vi "ClassPanel.vi"(8 "error in (no error)":errorcluster caption="entrée d'erreur (pas d'erreur)", 11 "E8267D.lvclass":refnum<class "E8267D.lvclass">) -> (0 "error out":errorcluster caption="sortie d'erreur", 3 "E8267D.lvclass Out":refnum<class "E8267D.lvclass">)   [LabVIEW 2019, in "E8267D.lvclass"]
uses:
  E8267D.lvclass
  C:/Programmes Labview/LabscanV1A/DevicesClass/BaseDevice/BaseDevice.lvclass
  BaseDevice/ClassQueueMess.ctl
  E8267D_Func.ctl
  E8267D.lvclass/E8267D.ctl
  BaseDevice/Accessor/GetClassEvent.vi
panel:
  in  "PulseMode En":bool
  in  "Mod En":bool
  in  "Scan Mode":u16(ring) items=["Frequency", "Power"]
  in  "Output En":bool
  in  "Con/Disc.":bool
  in  "FUnits":u16(ring) caption="Units" items=["Hz", "MHz", "GHz"]
  in  "MainProgQ":refnum<queue>
  in  "MainProgQEvent":refnum<user-event>
  in  "Acq":bool
  in  "Stop":bool
  in  "Power":dbl caption="Power(dBm)" format="%#.3f"
  in  "MiseAJour":bool
  in  "Freq(Hz)":dbl=60.0 min=0.01 max=20500000000.0 step=0.01 format="%^#.5e"
  out "Init Program":bool
  # "PSG E8267D"
  # "this MUST labeled with class name"
  # "this MUST be present and labeled \"Stop\" and \"Acq\""
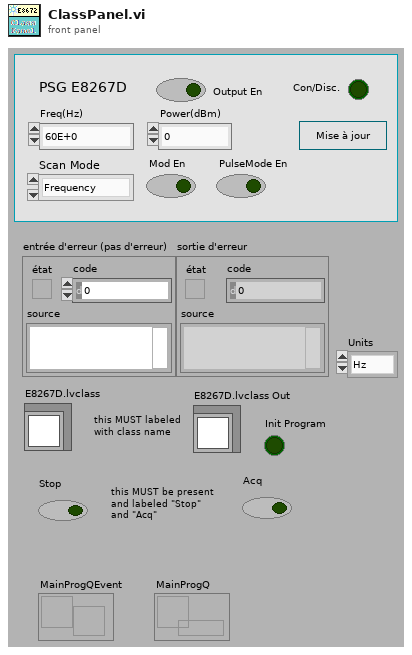
[diagram p1: front panel]
types:
  T1 = typedef "E8267D.lvclass/E8267D_Func.ctl" = enum16{"SetPower (dBm)", "SetFrequency (Hz)"}
  T2 = typedef "ClassQueueMess.ctl" = u16
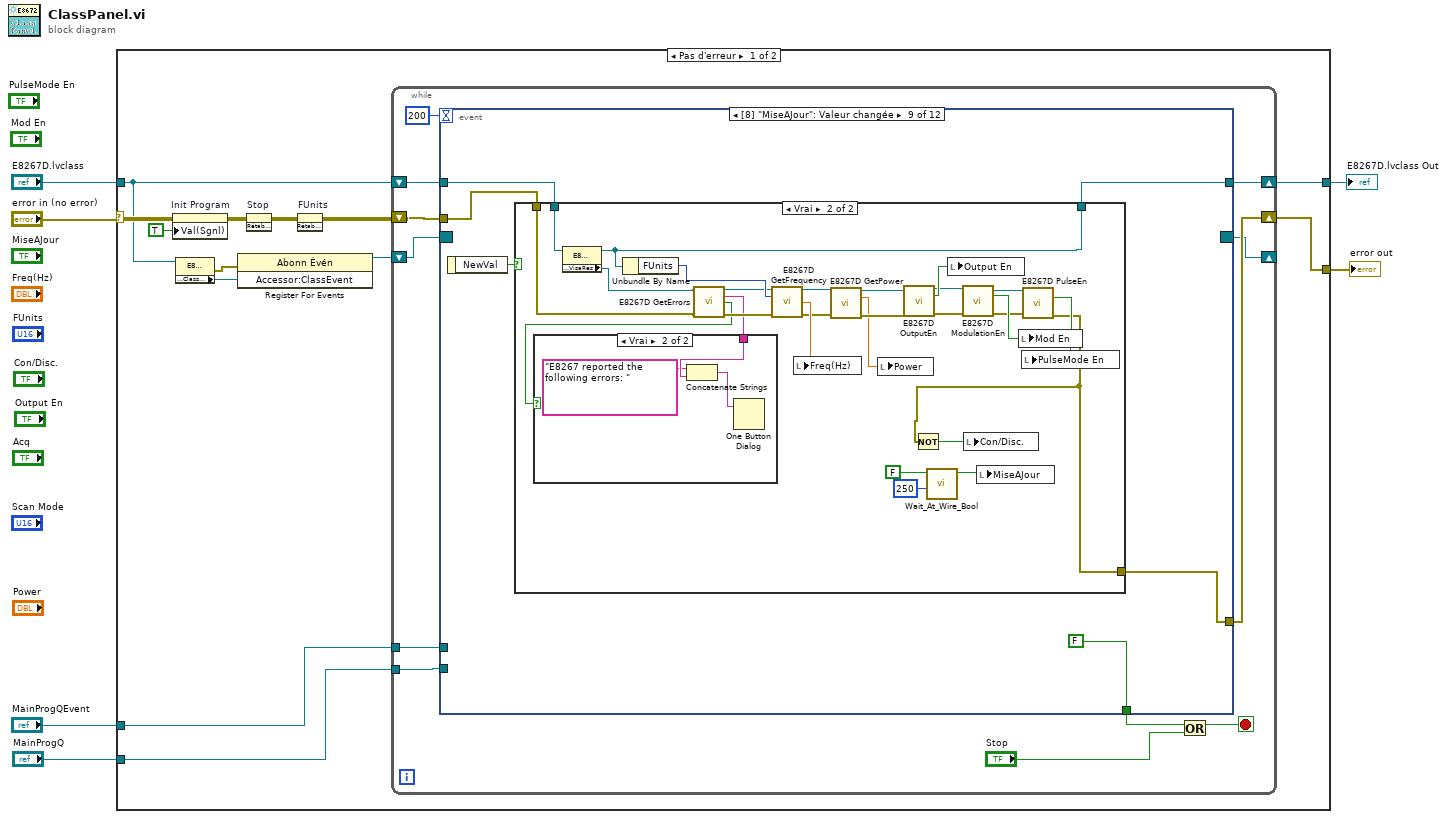
[diagram p0: block diagram]
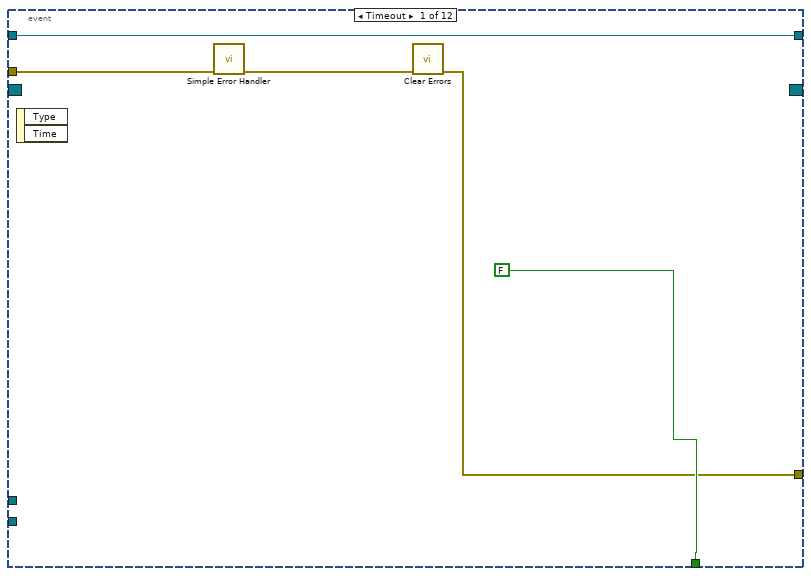
[diagram p2: hidden frame]
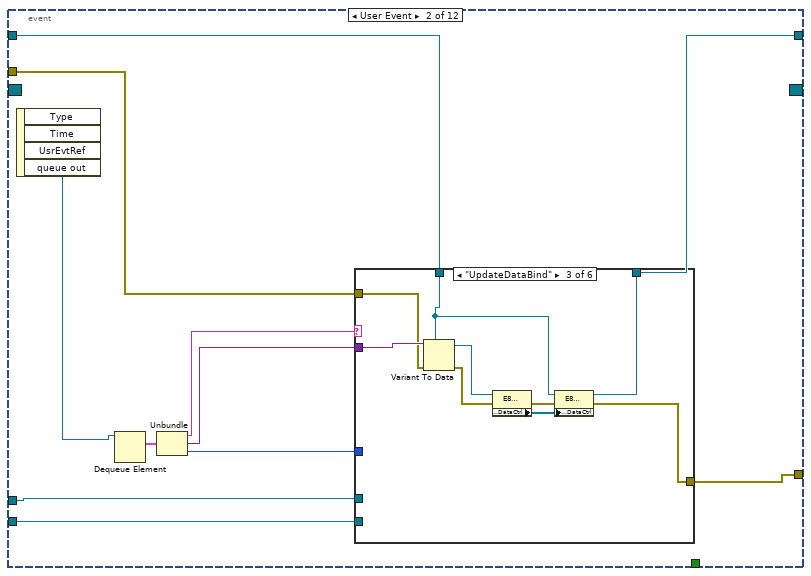
[diagram p3: hidden frame]
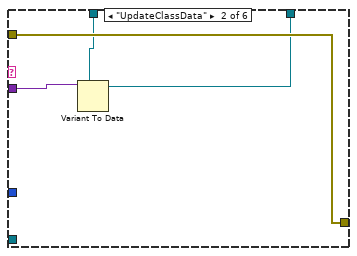
[diagram p5: hidden frame]
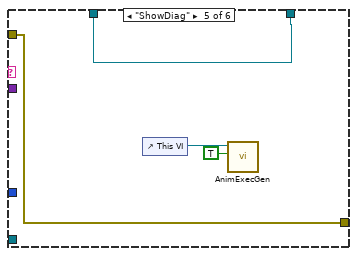
[diagram p7: hidden frame]
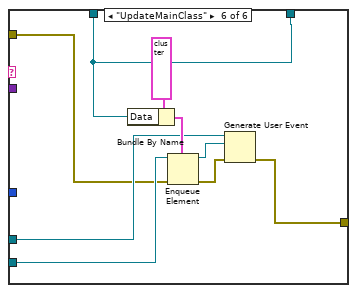
[diagram p8: hidden frame]
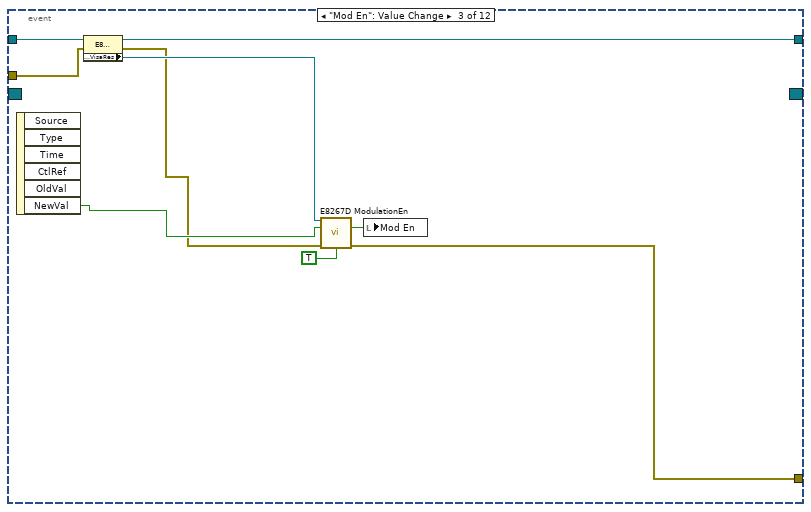
[diagram p9: hidden frame]
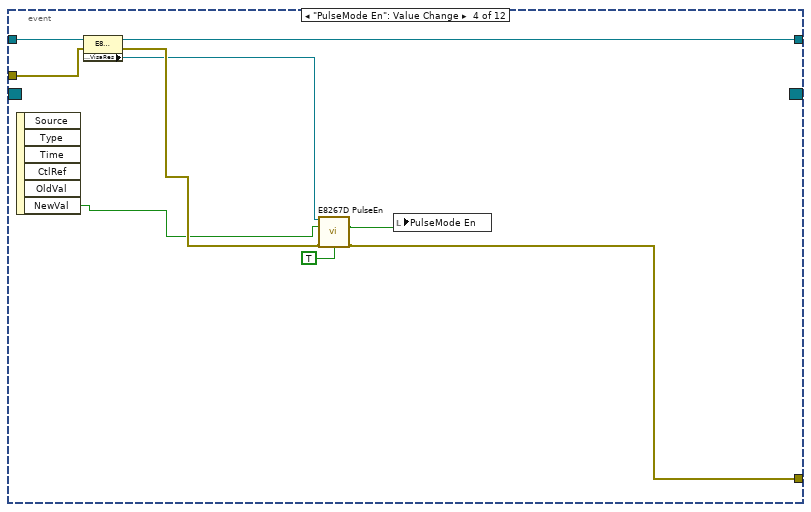
[diagram p10: hidden frame]
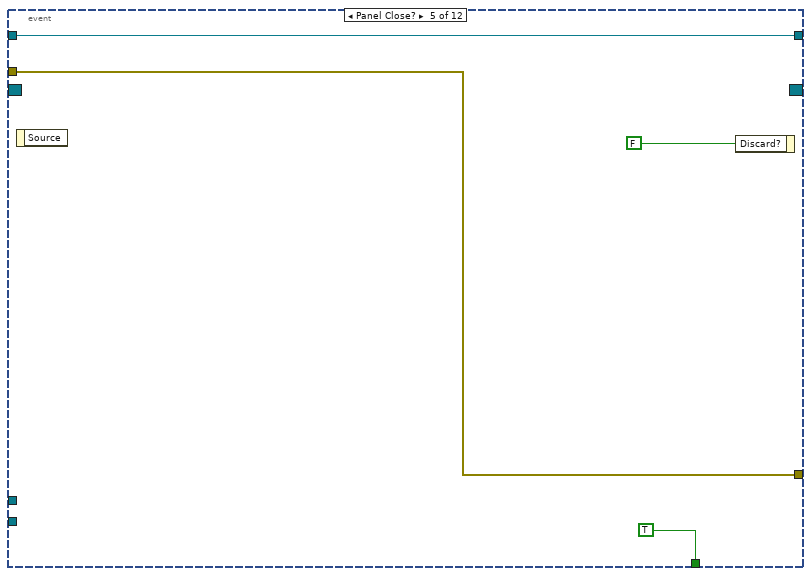
[diagram p11: hidden frame]
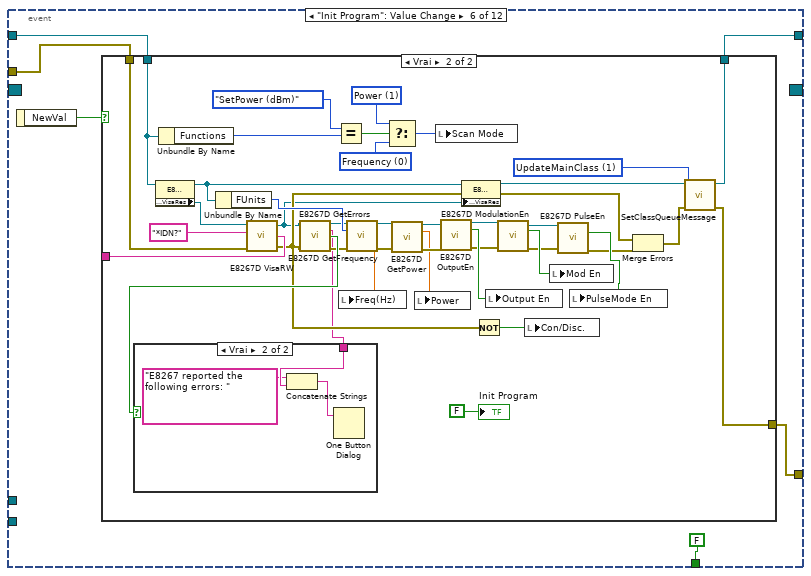
[diagram p12: hidden frame]
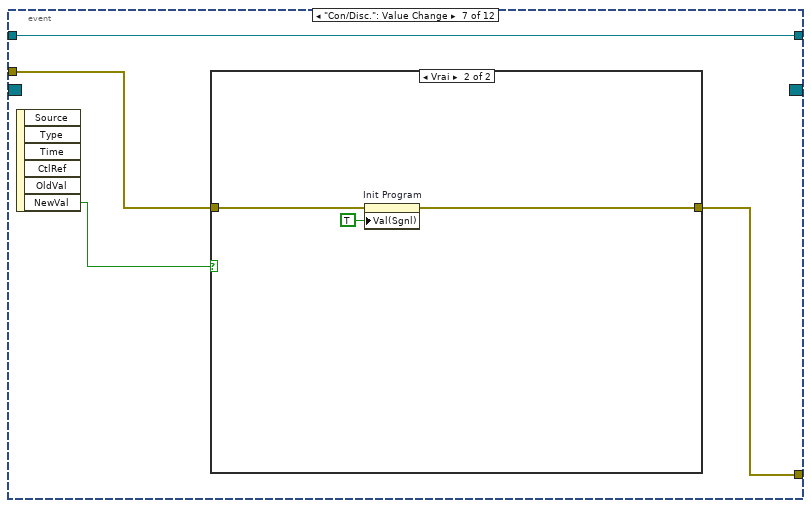
[diagram p15: hidden frame]
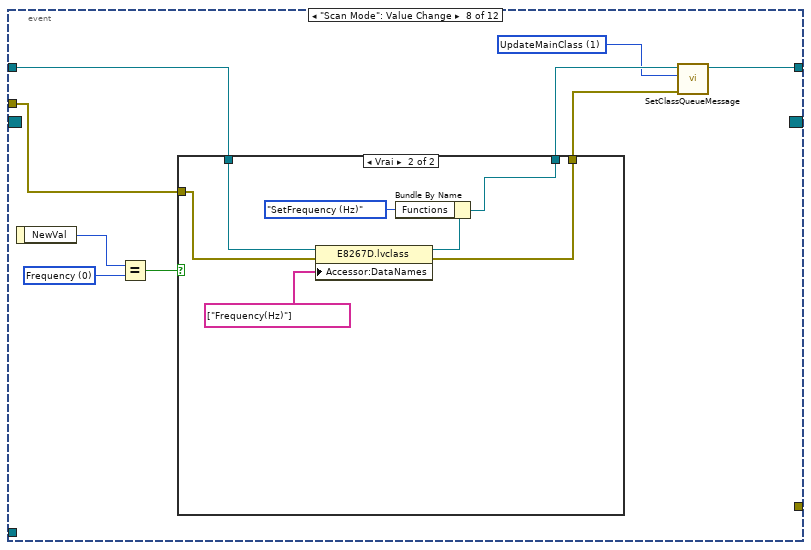
[diagram p17: hidden frame]
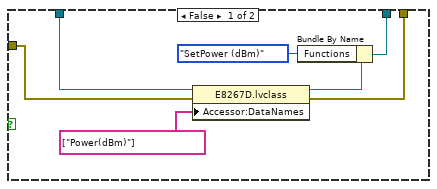
[diagram p18: hidden frame]
diagram:
  n1 = case shown="Pas d'erreur" "error in (no error)" {
    selector: "error in (no error)" -> [w16 w249]
    tunnel: [w19 w249] -> w5
    tunnel: "E8267D.lvclass" -> [w12 w248]
    tunnel: [w17 w248] -> w3
    tunnel: "MainProgQEvent" -> [w10 _]
    tunnel: "MainProgQ" -> [w9 _]
    frame No Error {
      n2 = property on="Init Program" class="Bool (strict)"(error in=w16, "Val(Sgnl)"=TRUE ("Valeur (Signalisation)")) -> (error out=w15:errorcluster)  [unwired: 1 in, 1 out]
      n3 = property class="E8267D.lvclass"(reference=w12) -> (error out=w14:errorcluster, "Accessor:ClassEvent"=w13:refnum<user-event>)  [unwired: 1 in, 1 out]
      n4 = register-events(error in=w14, w13) -> (reference out=w11:refnum<event-registration>)  [unwired: 1 in, 1 out]
      n5 = invoke on="Stop" class="Bool (strict)" method="RétablirValParDéfaut"(error in=w15) -> (error out=w8:errorcluster)  [unwired: 2 in, 2 out]
      n6 = invoke on="FUnits" class="MDér (strict)" method="RétablirValParDéfaut"(error in=w8) -> (error out=w7:errorcluster)  [unwired: 2 in, 2 out]
      n7 = while {
        shift-right: [w29] -> w19
        shift-left: w7 -> [w30]
        shift-right: [w26] -> w17
        shift-left: w12 -> [w28]
        shift-right: [w22] -> _
        shift-left: w11 -> [w23]
        tunnel: w10 -> [w21]
        tunnel: w9 -> [w20]
        stop <- w25 stop-if-true
        n8 = event shown="[8] \"MiseAJour\": Valeur changée" {
          selector: w23 -> [_ _ _ _ _ _ _ _ _ _ _ _]
          dyn-events: [_ _ _ _ _ _ _ _ _ _ _ _] -> w22
          timeout: 200 -> [_ _ _ _ _ _ _ _ _ _ _ _]
          tunnel: w30 -> [w34 w46 w82 w93 w97 w104 w153 w162 w187 w228 _ _]
          tunnel: [w32 w40 w80 w92 w97 w103 w152 _ w186 w222 w236 w245] -> w29
          tunnel: w28 -> [w35 w47 w85 w95 w96 w101 w155 w164 w184 w230 w239 w247]
          tunnel: [FALSE _ _ _ TRUE FALSE _ _ FALSE _ _ _] -> w27
          tunnel: [w35 w39 w84 w94 w96 w100 w155 w165 w183 w229 w238 w246] -> w26
          tunnel: w21 -> [_ w38 _ _ _ _ _ _ _ _ _ _]
          tunnel: w20 -> [_ w37 _ _ _ _ _ _ _ _ _ _]
          event Timeout {
            n9 = event-data() -> ()  [unwired: 1 in, 2 out]
            n10 = call <vilib>:"Simple Error Handler.vi"("error in (no error)"=w34) -> ("error out"=w33:errorcluster)  [unwired: 4 in, 4 out]
            n11 = call <vilib>:"Clear Errors.vi"("error in (no error)"=w33) -> ("error out"=w32:errorcluster)  [unwired: 5 in, 1 out]
          }
          event User Event {
            n12 = event-data() -> ("queue out"=w44:refnum<queue>)  [unwired: 1 in, 3 out]
            n13 = Dequeue Element(queue=w44) -> (element=w45:cluster{"Message":string, "Data":variant, i32})  [unwired: 2 in, 3 out]
            n14 = Unbundle(w45) -> ("Message"=w43:string, "Data"=w42:variant, w41:i32)
            n15 = case shown="\"UpdateDataBind\"" w43 {
              tunnel: w46 -> [w49 w53 w57 w63 w67 w70]
              tunnel: w42 -> [_ w52 w62 _ _ _]
              tunnel: w47 -> [w48 w51 w54 w64 w68 w73]
              tunnel: [w48 w50 w55 w64 w68 w73] -> w39
              tunnel: [w49 w53 w56 w63 w67 w69] -> w40
              tunnel: w41 -> [_ _ _ _ _ _]
              tunnel: w38 -> [_ _ _ _ _ w72]
              tunnel: w37 -> [_ _ _ _ _ w71]
              frame Default {
              }
              frame "UpdateClassData" {
                n16 = Variant To Data(type=w51, Variant=w52) -> (data=w50:refnum<class "E8267D.lvclass">)  [unwired: 1 in, 1 out]
              }
              frame "UpdateDataBind" {
                n17 = Variant To Data(error in=w57, type=w54, Variant=w62) -> (data=w59:refnum<class "E8267D.lvclass">, error out=w58:errorcluster)
                n18 = property class="E8267D.lvclass"(reference=w59, error in=w58) -> (error out=w61:errorcluster, "Accessor:DataCtrl"=w60:refnum<vi>[])  [unwired: 1 out]
                n19 = property class="E8267D.lvclass"(reference=w54, error in=w61, "Accessor:DataCtrl"=w60) -> (reference out=w55:refnum<class "E8267D.lvclass">, error out=w56:errorcluster)
              }
              frame "MeasDone" {
              }
              frame "ShowDiag" {
                n20 = control-ref of="This VI"() -> (w66:refnum<vi>)
                n21 = call <userlib>:"AnimExecGen.vi"("Animer l'exécution ?"=TRUE, "ViRef"=w66) -> ()  [unwired: 9 in, 1 out]
              }
              frame "UpdateMainClass" {
                n22 = Bundle By Name(cluster=cluster{"Message":string, "Data":variant, i32} {"Message"="", "Data"=variant, 0} ("élément"), "Data"=w73) -> (w74:cluster{"Message":string, "Data":variant, i32})
                n23 = Enqueue Element(queue=w71, element=w74, error in (no error)=w70) -> (queue out=w77:refnum<queue>, error out=w76:errorcluster)  [unwired: 1 in, 1 out]
                n24 = Generate User Event(user event=w72, event data cluster=w77, error in=w76) -> (error out=w69:errorcluster)  [unwired: 1 in, 1 out]
              }
            }
          }
          event "Mod En": Value Change {
            n25 = event-data() -> ("NewVal"=w86:bool)  [unwired: 1 in, 5 out]
            n26 = property class="E8267D.lvclass"(reference=w85, error in=w82) -> (reference out=w84:refnum<class "E8267D.lvclass">, error out=w81:errorcluster, "Accessor:VisaRes"=w83:refnum<visa-resource-name>)
            n27 = call <userlib>:"E8267D ModulationEn.vi"("VISA Rsrc"=w83, "Modulation En"=w86, "error in (no error)"=w81, "Set?(F)"=TRUE) -> ("Enabled"=w78:bool, "error out"=w80:errorcluster)  [unwired: 9 in, 1 out]
            n28 = local write "Mod En"(w78) -> ()
          }
          event "PulseMode En": Value Change {
            n29 = event-data() -> ("NewVal"=w90:bool)  [unwired: 1 in, 5 out]
            n30 = property class="E8267D.lvclass"(reference=w95, error in=w93) -> (reference out=w94:refnum<class "E8267D.lvclass">, error out=w91:errorcluster, "Accessor:VisaRes"=w89:refnum<visa-resource-name>)
            n31 = call <userlib>:"E8267D PulseEn.vi"("VISA Rsrc"=w89, "Modulation En"=w90, "error in (no error)"=w91, "Set?(F)"=TRUE) -> ("Enabled"=w87:bool, "error out"=w92:errorcluster)  [unwired: 9 in, 1 out]
            n32 = local write "PulseMode En"(w87) -> ()
          }
          event Panel Close? {
            n33 = event-data() -> ()  [unwired: 1 in, 1 out]
            n34 = event-data("Discard?"=FALSE ("Rejeter ?")) -> ()  [unwired: 1 in, 1 out]
          }
          event "Init Program": Value Change {
            n35 = event-data() -> ("NewVal"=w105:bool)  [unwired: 1 in]
            n36 = case shown="Vrai" w105 {
              tunnel: w104 -> [w107 w146]
              tunnel: [w107 w135] -> w103
              tunnel: w101 -> [w106 w128]
              tunnel: [w106 w140] -> w100
              tunnel: [_ w121] -> _
              frame False {
              }
              frame True {
                w122 = u16 0 items=["Frequency", "Power"] ("Scan Mode")
                w123 = u16 1 items=["Frequency", "Power"] ("Scan Mode")
                w139 = T2 1 items=["UpdateClassData", "UpdateMainClass", "UpdateDataBind", "ReInitDevice", "Custom", "ClosePan"] ("Menu déroulant")
                n37 = property class="E8267D.lvclass"(reference=w128) -> (reference out=w142:refnum<class "E8267D.lvclass">, "Accessor:VisaRes"=w147:refnum<visa-resource-name>)  [unwired: 1 in, 1 out]
                n38 = Unbundle By Name(w128) -> ("Functions"=w126:T1)
                n39 = Unbundle By Name(w142) -> ("FUnits"=w141:u16)
                n40 = call <userlib>:"E8267D VisaRW.vi"("error in (no error)"=w146, "ChaineCom"="*IDN?", "VISA Rsrc"=w147) -> ("error out"=w111:errorcluster, "ChaineRep"=w121:string, "VISA Rsrc Out"=w109:refnum<visa-resource-name>)  [unwired: 4 in, 1 out]
                n41 = call <userlib>:"E8267D GetErrors.vi"("VISA Rsrc"=w109, "error in (no error)"=w111) -> ("VISA Rsrc Out"=w113:refnum<visa-resource-name>, "Err String"=w108:string, "Errors"=w112:bool, "error out"=w110:errorcluster)  [unwired: 10 in]
                n42 = case shown="Vrai" w112 {
                  tunnel: w108 -> [_ w151]
                  frame False {
                  }
                  frame True {
                    n43 = Concatenate Strings("E8267 reported the following errors: " ("chaîne"), w151) -> (w150:string)
                    n44 = One Button Dialog(message=w150) -> ()  [unwired: 1 in, 1 out]
                  }
                }
                n45 = Equal?(x=E8267D_Func."SetPower (dBm)" ("Functions"), y=w126) -> (x = y?=w125:bool)
                n46 = call <userlib>:"E8267D GetFrequency.vi"("VISA Rsrc"=w113, "FUnits"=w141, "error in (no error)"=w110) -> ("VISA Rsrc Out"=w133:refnum<visa-resource-name>, "Frequency (Units)"=w143:dbl, "error out"=w134:errorcluster)  [unwired: 9 in, 1 out]
                n47 = local write "Freq(Hz)"(w143) -> ()
                n48 = Select(t=w123, s=w125, f=w122) -> (s? t:f=w124:u16)
                n49 = call <userlib>:"E8267D GetPower.vi"("VISA Rsrc"=w133, "error in (no error)"=w134) -> ("VISA Rsrc Out"=w130:refnum<visa-resource-name>, "Power (dBm)"=w131:dbl, "error out"=w132:errorcluster)  [unwired: 11 in]
                n50 = local write "Power"(w131) -> ()
                n51 = local write "Scan Mode"(w124) -> ()
                n52 = call <userlib>:"E8267D OutputEn.vi"("VISA Rsrc"=w130, "error in (no error)"=w132) -> ("VISA Rsrc Out"=w118:refnum<visa-resource-name>, "Enabled"=w129:bool, "error out"=w119:errorcluster)  [unwired: 11 in]
                n53 = property class="E8267D.lvclass"(reference=w142, error in=w111, "Accessor:VisaRes"=w109) -> (reference out=w138:refnum<class "E8267D.lvclass">, error out=w137:errorcluster)
                n54 = Not(x=w111) -> (.not. x?=w144:bool)
                n55 = local write "Output En"(w129) -> ()
                n56 = call <userlib>:"E8267D ModulationEn.vi"("VISA Rsrc"=w118, "error in (no error)"=w119) -> ("VISA Rsrc Out"=w116:refnum<visa-resource-name>, "Enabled"=w120:bool, "error out"=w117:errorcluster)  [unwired: 11 in]
                n57 = local write "Con/Disc."(w144) -> ()
                n58 = local write "Mod En"(w120) -> ()
                n59 = call <userlib>:"E8267D PulseEn.vi"("VISA Rsrc"=w116, "error in (no error)"=w117) -> ("Enabled"=w115:bool, "error out"=w114:errorcluster)  [unwired: 11 in, 1 out]
                n60 = local write "PulseMode En"(w115) -> ()
                n61 = Merge Errors(w137, w114) -> (w136:errorcluster)
                n62 = call-dynamic "SetClassQueueMessage.vi"("ErrorIn(No Error)"=w136, "Menu déroulant"=w139, "DefaultDev.lvclass"=w138) -> ("sortie d'erreur"=w135:errorcluster, "DefaultDev.lvclass Out"=w140:refnum<class "E8267D.lvclass">)  [unwired: 7 in]
                "Init Program" <- FALSE
              }
            }
          }
          event "Con/Disc.": Value Change {
            n63 = event-data() -> ("NewVal"=w154:bool)  [unwired: 1 in, 5 out]
            n64 = case shown="Vrai" w154 {
              tunnel: w153 -> [w156 w158]
              tunnel: [w156 w157] -> w152
              frame False {
              }
              frame True {
                n65 = property on="Init Program" class="Bool (strict)"(error in=w158, "Val(Sgnl)"=TRUE ("Valeur (Signalisation)")) -> (error out=w157:errorcluster)  [unwired: 1 in, 1 out]
              }
            }
          }
          event "Scan Mode": Value Change {
            w160 = T2 1 items=["UpdateClassData", "UpdateMainClass", "UpdateDataBind", "ReInitDevice", "Custom", "ClosePan"] ("Menu déroulant")
            w168 = u16 0 items=["Frequency", "Power"] ("Scan Mode")
            n66 = event-data() -> ("NewVal"=w167:u16)  [unwired: 1 in]
            n67 = Equal?(x=w167, y=w168) -> (x = y?=w166:bool)
            n68 = case shown="Vrai" w166 {
              tunnel: w164 -> [w173 w180]
              tunnel: [w174 w181] -> w163
              tunnel: w162 -> [w170 w179]
              tunnel: [w169 w178] -> w161
              frame False {
                n69 = property class="E8267D.lvclass"(reference=w173, error in=w170, "Accessor:DataNames"=string[] ["Power(dBm)"]) -> (reference out=w172:refnum<class "E8267D.lvclass">, error out=w169:errorcluster)
                n70 = Bundle By Name(cluster=w172, "Functions"=E8267D_Func."SetPower (dBm)") -> (w174:refnum<class "E8267D.lvclass">)
              }
              frame True {
                n71 = property class="E8267D.lvclass"(reference=w180, error in=w179, "Accessor:DataNames"=string[] ["Frequency(Hz)"]) -> (reference out=w177:refnum<class "E8267D.lvclass">, error out=w178:errorcluster)
                n72 = Bundle By Name(cluster=w177, "Functions"=E8267D_Func."SetFrequency (Hz)") -> (w181:refnum<class "E8267D.lvclass">)
              }
            }
            n73 = call-dynamic "SetClassQueueMessage.vi"("ErrorIn(No Error)"=w161, "Menu déroulant"=w160, "DefaultDev.lvclass"=w163) -> ("DefaultDev.lvclass Out"=w165:refnum<class "E8267D.lvclass">)  [unwired: 7 in, 1 out]
          }
          event "MiseAJour": Value Change {
            n74 = event-data() -> ("NewVal"=w188:bool)  [unwired: 1 in]
            n75 = case shown="Vrai" w188 {
              tunnel: w187 -> [w190 w202]
              tunnel: [w190 w192] -> w186
              tunnel: w184 -> [w189 w217]
              tunnel: [w189 w205] -> w183
              frame False {
              }
              frame True {
                n76 = property class="E8267D.lvclass"(reference=w217) -> (reference out=w205:refnum<class "E8267D.lvclass">, "Accessor:VisaRes"=w201:refnum<visa-resource-name>)  [unwired: 1 in, 1 out]
                n77 = Unbundle By Name(w205) -> ("FUnits"=w214:u16)
                n78 = call <userlib>:"E8267D GetErrors.vi"("VISA Rsrc"=w201, "error in (no error)"=w202) -> ("VISA Rsrc Out"=w191:refnum<visa-resource-name>, "Err String"=w200:string, "Errors"=w199:bool, "error out"=w203:errorcluster)  [unwired: 10 in]
                n79 = case shown="Vrai" w199 {
                  tunnel: w200 -> [_ w220]
                  frame False {
                  }
                  frame True {
                    n80 = Concatenate Strings("E8267 reported the following errors: " ("chaîne"), w220) -> (w219:string)
                    n81 = One Button Dialog(message=w219) -> ()  [unwired: 1 in, 1 out]
                  }
                }
                n82 = call <userlib>:"E8267D GetFrequency.vi"("VISA Rsrc"=w191, "FUnits"=w214, "error in (no error)"=w203) -> ("VISA Rsrc Out"=w212:refnum<visa-resource-name>, "Frequency (Units)"=w215:dbl, "error out"=w213:errorcluster)  [unwired: 9 in, 1 out]
                n83 = local write "Freq(Hz)"(w215) -> ()
                n84 = call <userlib>:"E8267D GetPower.vi"("VISA Rsrc"=w212, "error in (no error)"=w213) -> ("VISA Rsrc Out"=w209:refnum<visa-resource-name>, "Power (dBm)"=w210:dbl, "error out"=w211:errorcluster)  [unwired: 11 in]
                n85 = local write "Power"(w210) -> ()
                n86 = call <userlib>:"E8267D OutputEn.vi"("VISA Rsrc"=w209, "error in (no error)"=w211) -> ("VISA Rsrc Out"=w194:refnum<visa-resource-name>, "Enabled"=w204:bool, "error out"=w193:errorcluster)  [unwired: 11 in]
                n87 = call <userlib>:"Wait_At_Wire_Bool.vi"("Wait (ms)"=u32 250, "error in (no error)"=FALSE) -> ("error out"=w207:bool)  [unwired: 7 in, 2 out]
                n88 = local write "Output En"(w204) -> ()
                n89 = call <userlib>:"E8267D ModulationEn.vi"("VISA Rsrc"=w194, "error in (no error)"=w193) -> ("VISA Rsrc Out"=w196:refnum<visa-resource-name>, "Enabled"=w198:bool, "error out"=w197:errorcluster)  [unwired: 11 in]
                n90 = local write "MiseAJour"(w207) -> ()
                n91 = local write "Mod En"(w198) -> ()
                n92 = call <userlib>:"E8267D PulseEn.vi"("VISA Rsrc"=w196, "error in (no error)"=w197) -> ("Enabled"=w195:bool, "error out"=w192:errorcluster)  [unwired: 11 in, 1 out]
                n93 = Not(x=w192) -> (.not. x?=w216:bool)
                n94 = local write "Con/Disc."(w216) -> ()
                n95 = local write "PulseMode En"(w195) -> ()
              }
            }
          }
          event "Freq(Hz)": Value Change {
            n96 = event-data() -> ("NewVal"=w226:dbl)  [unwired: 1 in, 5 out]
            n97 = property class="E8267D.lvclass"(reference=w230) -> (reference out=w229:refnum<class "E8267D.lvclass">, "Accessor:VisaRes"=w227:refnum<visa-resource-name>)  [unwired: 1 in, 1 out]
            n98 = local read "FUnits"() -> (w224:u16)
            n99 = call <userlib>:"E8267D SetFrequency.vi"("VISA Rsrc"=w227, "Frequency (Hz)"=w226, "FUnits"=w224, "error in (no error)"=w228) -> ("VISA Rsrc Out"=w225:refnum<visa-resource-name>, "error out"=w223:errorcluster)  [unwired: 10 in]
            n100 = call <userlib>:"E8267D GetFrequency.vi"("VISA Rsrc"=w225, "FUnits"=w224, "error in (no error)"=w223) -> ("Frequency (Hz)"=w221:dbl, "error out"=w222:errorcluster)  [unwired: 9 in, 2 out]
            n101 = local write "Freq(Hz)"(w221) -> ()
          }
          event "Power": Value Change {
            n102 = event-data() -> ("NewVal"=w231:dbl)  [unwired: 1 in, 5 out]
            n103 = property class="E8267D.lvclass"(reference=w239) -> (reference out=w238:refnum<class "E8267D.lvclass">, error out=w232:errorcluster, "Accessor:VisaRes"=w234:refnum<visa-resource-name>)  [unwired: 1 in]
            n104 = call <userlib>:"E8267D SetPower.vi"("VISA Rsrc"=w234, "Power dBm"=w231, "error in (no error)"=w232) -> ("VISA Rsrc Out"=w233:refnum<visa-resource-name>, "error out"=w235:errorcluster)  [unwired: 11 in]
            n105 = call <userlib>:"E8267D GetPower.vi"("VISA Rsrc"=w233, "error in (no error)"=w235) -> ("Power (dBm)"=w237:dbl, "error out"=w236:errorcluster)  [unwired: 11 in, 1 out]
            n106 = local write "Power"(w237) -> ()
          }
          event "Output En": Value Change {
            n107 = event-data() -> ("NewVal"=w242:bool)  [unwired: 1 in, 5 out]
            n108 = property class="E8267D.lvclass"(reference=w247) -> (reference out=w246:refnum<class "E8267D.lvclass">, error out=w243:errorcluster, "Accessor:VisaRes"=w244:refnum<visa-resource-name>)  [unwired: 1 in]
            n109 = call <userlib>:"E8267D OutputEn.vi"("VISA Rsrc"=w244, "Output En"=w242, "error in (no error)"=w243, "Set?(F)"=TRUE) -> ("Enabled"=w240:bool, "error out"=w245:errorcluster)  [unwired: 9 in, 1 out]
            n110 = local write "Output En"(w240) -> ()
          }
        }
        n111 = Or(x=w27, y="Stop") -> (x .or. y?=w25:bool)
      }
    }
    frame Error {
    }
  }
  "error out" <- w5
  "E8267D.lvclass Out" <- w3
